vi "Info.vi"(4 "Source":string, 6 "Message":string, 7 "Logger Name (Logger)":string="Logger", 8 "error in (no error)":errorcluster) -> (0 "error out":errorcluster)   [LabVIEW 2024, in "LogSingleton.lvlib"]
uses:
  LogSingleton.lvlib
  RQMHLogger/Logger.lvclass
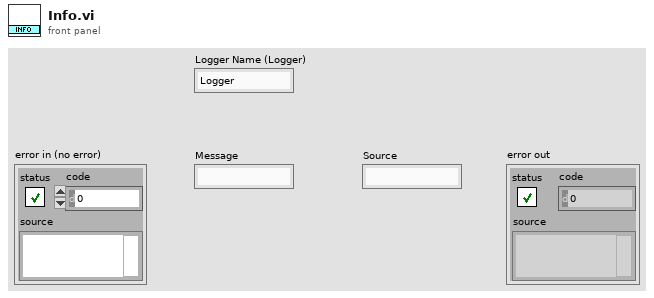
[diagram p1: front panel]
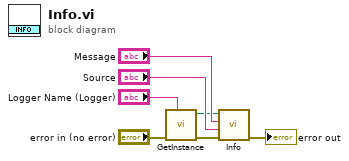
[diagram p0: block diagram]
diagram:
  n1 = call "GetInstance.vi"("Logger Name (Logger)"="Logger Name (Logger)", "error in (no error)"="error in (no error)") -> ("error out"=w2:errorcluster, "RQMHLogger Get"=w1:refnum<class "Logger.lvclass">)  [unwired: 8 in]
  n2 = call "Info.vi"("error in (no error)"=w2, "Source"="Source", "Message"="Message", "RQMHLogger in"=w1) -> ("error out"=→"error out":errorcluster)  [unwired: 6 in, 1 out]
